vi "Read All Form Data (LV2011).vi"(8 "error in (no error)":errorcluster, 11 "httpRequestID":u32) -> (0 "error out":errorcluster, 2 "form data":cluster{"Key":string[], "Value":string[]}, 3 "httpRequestID out":u32)   [LabVIEW 2020, in "NI_WebServices.lvlib"]
doc: "Reads the form data values received from the specified HTTP request. This VI processes that form data and assigns those values to elements in a 1D array. Use this VI for requests that use the multipart/form-data encoding type."
uses:
  <vilib>/wsapi/NI_WebServices.lvlib
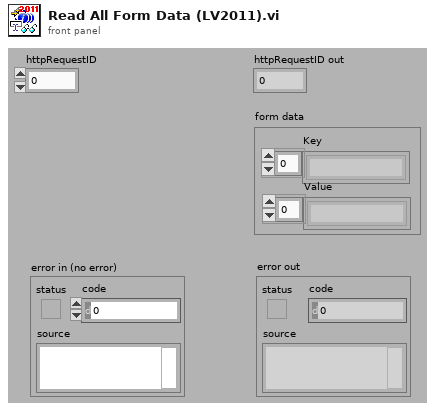
[diagram p1: front panel]
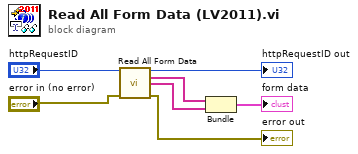
[diagram p0: block diagram]
diagram:
  n1 = call <vilib>:"Read All Form Data.vi"("httpRequestID"="httpRequestID", "error in (no error)"="error in (no error)") -> ("httpRequestID out"=→"httpRequestID out":u32, "Key"=w3:string[], "Value"=w2:string[], "error out"=→"error out":errorcluster)  [unwired: 9 in, 1 out]
  n2 = Bundle("Key"=w3, "Value"=w2) -> (→"form data":cluster{"Key":string[], "Value":string[]})  [unwired: 1 in]
